vi "Tektronix AFG 1000 Series Amplitude Modulation.vi"() -> ()   [LabVIEW 2016]
doc: "Demonstrates how to configure and generate an amplitude modulated waveform."
uses:
  Public/Configure/Configure Modulation (AM).vi
  Tektronix AFG 1000 Series.lvlib
panel:
  in  "Phase Unit (0: Radian)":u16(ring) items=["Radians", "Degrees"]
  in  "Phase (0)":dbl
  in  "Channel (1: Channel 1)":u16(ring)=1 items=["Channel 1"=1, "Channel 2"=2]
  in  "Modulation Frequency (100 Hz)":dbl=100.0
  in  "Modulation Depth (3 %)":dbl=3.0
  in  "Modulation Waveform (0: Sine)":u16(ring) items=["Sine", "Square", "Ramp", "Noise", "User Waveform", "Edit Memory", "EFile"]
  in  "Enable AM (T: Enable)":bool=TRUE
  in  "Amplitude (1 Vpp)":dbl=1.0
  in  "DC Offset (0.00 V)":dbl
  in  "Frequency (1000 Hz)":dbl=1000.0
  in  "Waveform Function (0: Sine)":u16(ring) items=["Sine", "Square", "Pulse", "Ramp", "Noise"]
  in  "VISA resource name":refnum<visa-resource-name>
  # "(c) 2016 National Instruments.  ALL RIGHTS RESERVED."
  # "Internal Settings"
  # "Carrier Settings"
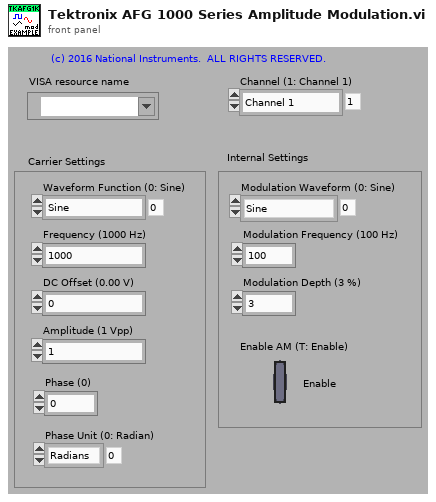
[diagram p1: front panel]
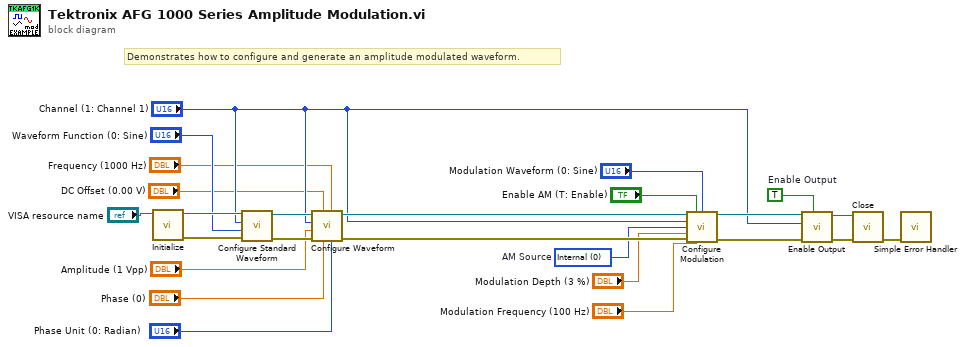
[diagram p0: block diagram]
diagram:
  w12 = TRUE  # Enable Output
  w15 = u16 0 items=["Internal", "External"]  # AM Source
  # "Demonstrates how to configure and generate an amplitude modulated waveform."
  n1 = call "Initialize.vi"("VISA resource name"="VISA resource name") -> ("error out"=w11:errorcluster, "VISA resource name out"=w9:refnum<visa-resource-name>)  [unwired: 9 in]
  n2 = call "Configure Standard Waveform.vi"("error in (no error)"=w11, "Waveform Function (0: Sine)"="Waveform Function (0: Sine)", "Channel (1 Channel 1)"="Channel (1: Channel 1)", "VISA resource name"=w9) -> ("error out"=w10:errorcluster, "VISA resource name out"=w8:refnum<visa-resource-name>)  [unwired: 6 in]
  n3 = call "Configure Waveform.vi"("Phase Unit (0: Radian)"="Phase Unit (0: Radian)", "Frequency (1000 Hz)"="Frequency (1000 Hz)", "Phase (0)"="Phase (0)", "DC Offset (0.00 V)"="DC Offset (0.00 V)", "error in (no error)"=w10, "Amplitude (1 Vpp)"="Amplitude (1 Vpp)", "Channel (1 Channel 1)"="Channel (1: Channel 1)", "VISA resource name"=w8) -> ("error out"=w18:errorcluster, "VISA resource name out"=w24:refnum<visa-resource-name>)  [unwired: 2 in]
  n4 = call-poly "Configure Modulation.vi"("VISA resource name"=w24, "Enable AM (T: Enable)"="Enable AM (T: Enable)", "Modulation Waveform (0: Sine)"="Modulation Waveform (0: Sine)", "Channel (1: Channel 1)"="Channel (1: Channel 1)", "AM Source (0: Internal)"=w15, "Modulation Depth (3 %)"="Modulation Depth (3 %)", "error in (no error)"=w18, "Modulation Frequency (100 Hz)"="Modulation Frequency (100 Hz)") -> ("VISA resource name out"=w23:refnum<visa-resource-name>, "error out"=w19:errorcluster)  [unwired: 6 in]
  n5 = call "Enable Output.vi"("Enable Output (T: Enable)"=w12, "error in (no error)"=w19, "Channel (1: Channel 1)"="Channel (1: Channel 1)", "VISA resource name"=w23) -> ("error out"=w20:errorcluster, "VISA resource name out"=w22:refnum<visa-resource-name>)  [unwired: 6 in]
  n6 = call "Close.vi"("error in (no error)"=w20, "VISA resource name"=w22) -> ("error out"=w21:errorcluster)  [unwired: 9 in]
  n7 = call <vilib>:"Simple Error Handler.vi"("error in (no error)"=w21) -> ()  [unwired: 4 in, 5 out]
